vi "post.vi"(8 "error in (no error)":errorcluster, 10 "build_spec":T1, 11 "lv-build-default in":refnum<class "lv-builder.lvclass">) -> (0 "error out":errorcluster, 3 "lv-build-default out":refnum<class "lv-builder.lvclass">)   [LabVIEW 2015, in "lv-builder.lvlib" / "lv-builder.lvclass"]
uses:
  lv-builder.lvclass
  lv-build/public/_controls/build_specification.ctl
  lv-build/public/_controls/build_type.ctl
  public/_controls/configuration.ctl
  private/_controls/post_action_lvlib.ctl
  private/_controls/post_action_zip.ctl
  private/_controls/post_action_application.ctl
  private/_controls/post_action_installer.ctl
  lv-builder.lvlib
  lv-build/lv-build.lvlib
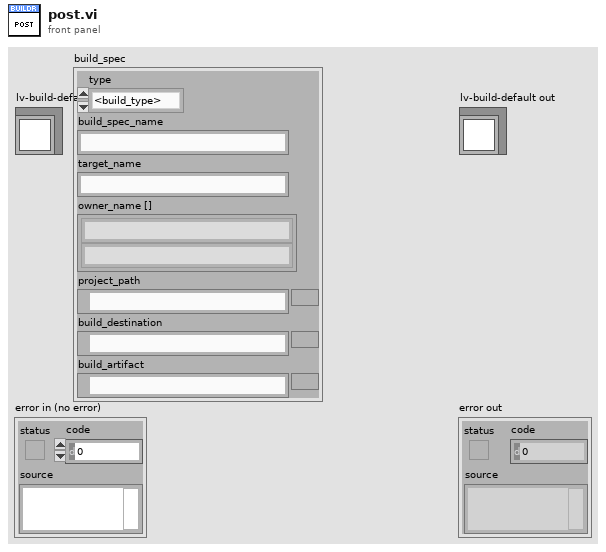
[diagram p1: front panel]
types:
  T1 = typedef "lv-build.lvlib/build_specification.ctl" = cluster{"type":T2, "build_spec_name":string, "target_name":string, "owner_name []":string[], "project_path":path, "build_destination":path, "build_artifact":path}
  T2 = typedef "lv-build.lvlib/build_type.ctl" = enum16{"<build_type>", "application_pc", "application_rt", "installer", "llb", "lvlibp", "zip", "fpga", "<null>"}
  T3 = typedef "lv-builder.lvlib/configuration.ctl" = cluster{"lvlibp_directory":string, "zip_directory":string, "lvlib_directory":string, "update_version_vi":string, "installer_post_file":string, "lvlib_post_action":u16, "installer_post_action":u16, "application_post_action":u16, "zip_post_action":u16}
  T4 = typedef "lv-builder.lvlib/post_action_lvlib.ctl" = enum16{"<lvlib_post_action>", "nothing", "move", "install", "<null>"}
  T5 = typedef "lv-builder.lvlib/post_action_zip.ctl" = enum16{"<zip_post_action>", "nothing", "move", "extract", "<null>"}
  T6 = typedef "lv-builder.lvlib/post_action_application.ctl" = enum16{"<application_post_action>", "nothing", "zip_application", "<null>"}
  T7 = typedef "lv-builder.lvlib/post_action_installer.ctl" = enum16{"<installer_post_action>", "nothing", "create_installer", "zip_installer", "create_installer_file", "<null>"}
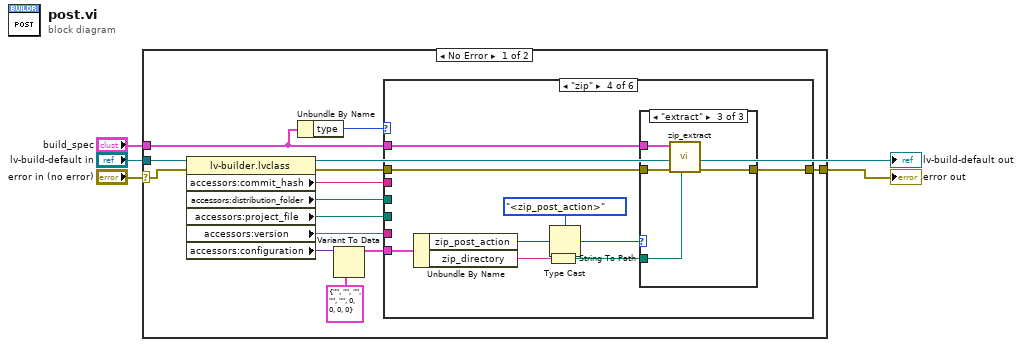
[diagram p0: block diagram]
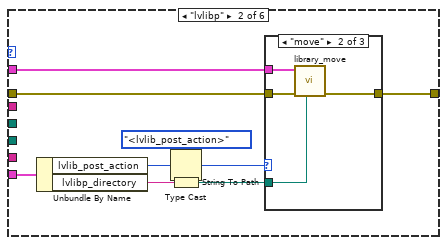
[diagram p3: hidden frame]
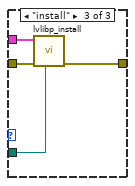
[diagram p5: hidden frame]
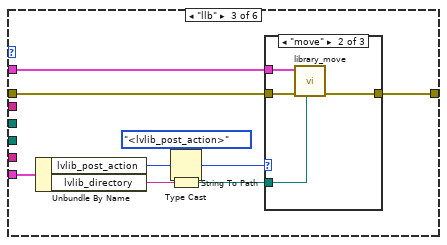
[diagram p6: hidden frame]
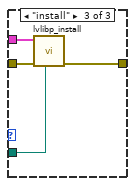
[diagram p8: hidden frame]
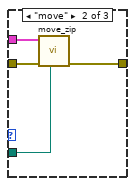
[diagram p10: hidden frame]
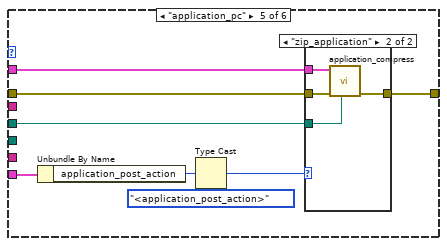
[diagram p11: hidden frame]
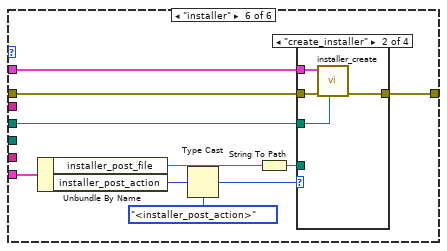
[diagram p13: hidden frame]
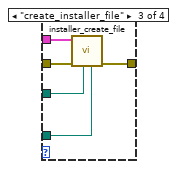
[diagram p15: hidden frame]
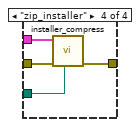
[diagram p16: hidden frame]
diagram:
  n1 = case shown="No Error" "error in (no error)" {
    selector: "error in (no error)" -> [w14 w110]
    tunnel: [w17 w110] -> w4
    tunnel: "build_spec" -> [w16 _]
    tunnel: "lv-build-default in" -> [w13 _]
    frame No Error {
      n2 = property class="lv-builder.lvclass"(reference=w13, error in=w14) -> (error out=w12:errorcluster, "accessors:commit_hash"=w11:string, "accessors:distribution_folder"=w10:path, "accessors:project_file"=w7:path, "accessors:version"=w9:string, "accessors:configuration"=w8:variant)  [unwired: 1 out]
      n3 = Unbundle By Name(w16) -> ("type"=w15:T2)
      n4 = Variant To Data(type=T3 {"lvlibp_directory"="", "zip_directory"="", "lvlib_directory"="", "update_version_vi"="", "installer_post_file"="", "lvlib_post_action"=0, "installer_post_action"=0, "application_post_action"=0, "zip_post_action"=0} ("configuration"), Variant=w8) -> (data=w5:T3)  [unwired: 1 in, 1 out]
      n5 = case shown="\"zip\"" w15 {
        tunnel: [w18 w27 w45 w63 w80 w95] -> w17
        tunnel: w16 -> [_ w26 w44 w62 w79 w94]
        tunnel: w12 -> [w18 w25 w43 w61 w78 w93]
        tunnel: w11 -> [_ _ _ _ _ _]
        tunnel: w10 -> [_ _ _ _ w73 w86]
        tunnel: w9 -> [_ _ _ _ _ _]
        tunnel: w5 -> [_ w21 w39 w57 w74 w91]
        tunnel: w7 -> [_ _ _ _ _ _]
        frame Default {
        }
        frame "lvlibp" {
          n6 = Unbundle By Name(w21) -> ("lvlib_post_action"=w23:u16, "lvlibp_directory"=w20:string)
          n7 = Type Cast(type=post_action_lvlib."<lvlib_post_action>" ("lvlib_post_action"), x=w23) -> (*(type *) &x=w22:T4)
          n8 = String To Path(string=w20) -> (path=w19:path)
          n9 = case shown="\"move\"" w22 {
            tunnel: [w28 w30 w34] -> w27
            tunnel: w26 -> [_ w31 w36]
            tunnel: w25 -> [w28 w32 w35]
            tunnel: w19 -> [_ w29 w33]
            frame Default {
            }
            frame "move" {
              n10 = call "library_move.vi"("lvlib_move_directory"=w29, "error in (no error)"=w32, "build_specifications"=w31) -> ("error out"=w30:errorcluster)  [unwired: 8 in]
            }
            frame "install" {
              n11 = call "lvlibp_install.vi"("lvlib_move_directory"=w33, "error in (no error)"=w35, "build_specifications"=w36) -> ("error out"=w34:errorcluster)  [unwired: 8 in]
            }
          }
        }
        frame "llb" {
          n12 = Unbundle By Name(w39) -> ("lvlib_post_action"=w41:u16, "lvlib_directory"=w38:string)
          n13 = Type Cast(type=post_action_lvlib."<lvlib_post_action>" ("lvlib_post_action"), x=w41) -> (*(type *) &x=w40:T4)
          n14 = String To Path(string=w38) -> (path=w37:path)
          n15 = case shown="\"move\"" w40 {
            tunnel: [w46 w48 w52] -> w45
            tunnel: w44 -> [_ w49 w54]
            tunnel: w43 -> [w46 w50 w53]
            tunnel: w37 -> [_ w47 w51]
            frame Default {
            }
            frame "move" {
              n16 = call "library_move.vi"("lvlib_move_directory"=w47, "error in (no error)"=w50, "build_specifications"=w49) -> ("error out"=w48:errorcluster)  [unwired: 8 in]
            }
            frame "install" {
              n17 = call "lvlibp_install.vi"("lvlib_move_directory"=w51, "error in (no error)"=w53, "build_specifications"=w54) -> ("error out"=w52:errorcluster)  [unwired: 8 in]
            }
          }
        }
        frame "zip" {
          n18 = Unbundle By Name(w57) -> ("zip_post_action"=w60:u16, "zip_directory"=w56:string)
          n19 = String To Path(string=w56) -> (path=w55:path)
          n20 = Type Cast(type=post_action_zip."<zip_post_action>" ("zip_post_action"), x=w60) -> (*(type *) &x=w59:T5)
          n21 = case shown="\"extract\"" w59 {
            tunnel: [w64 w66 w70] -> w63
            tunnel: w62 -> [_ w67 w71]
            tunnel: w61 -> [w64 w68 w72]
            tunnel: w55 -> [_ w65 w69]
            frame Default {
            }
            frame "move" {
              n22 = call "move_zip.vi"("zip_move_directory"=w65, "error in (no error)"=w68, "build_specifications"=w67) -> ("error out"=w66:errorcluster)  [unwired: 8 in]
            }
            frame "extract" {
              n23 = call "zip_extract.vi"("zip_extract_directory"=w69, "error in (no error)"=w72, "build_specifications"=w71) -> ("error out"=w70:errorcluster)  [unwired: 8 in]
            }
          }
        }
        frame "application_pc" {
          n24 = Unbundle By Name(w74) -> ("application_post_action"=w76:u16)
          n25 = Type Cast(type=post_action_application."<application_post_action>" ("application_post_action"), x=w76) -> (*(type *) &x=w75:T6)
          n26 = case shown="\"zip_application\"" w75 {
            tunnel: [w81 w83] -> w80
            tunnel: w79 -> [_ w85]
            tunnel: w78 -> [w81 w84]
            tunnel: w73 -> [_ w82]
            frame "nothing", Default {
            }
            frame "zip_application" {
              n27 = call "application_compress.vi"("distribution_folder"=w82, "error in (no error)"=w84, "build_specifications"=w85) -> ("error out"=w83:errorcluster)  [unwired: 8 in]
            }
          }
        }
        frame "installer" {
          n28 = Unbundle By Name(w91) -> ("installer_post_file"=w87:string, "installer_post_action"=w88:u16)
          n29 = Type Cast(type=post_action_installer."<installer_post_action>" ("installer_post_action"), x=w88) -> (*(type *) &x=w89:T7)
          n30 = String To Path(string=w87) -> (path=w92:path)
          n31 = case shown="\"create_installer\"" w89 {
            tunnel: [w96 w98 w103 w107] -> w95
            tunnel: w94 -> [_ w99 w104 w109]
            tunnel: w93 -> [w96 w100 w105 w108]
            tunnel: w92 -> [_ _ w101 _]
            tunnel: w86 -> [_ w97 w102 w106]
            frame "nothing", Default {
            }
            frame "create_installer" {
              n32 = call "installer_create.vi"("distribution_folder"=w97, "error in (no error)"=w100, "build_specifications"=w99) -> ("error out"=w98:errorcluster)  [unwired: 8 in]
            }
            frame "create_installer_file" {
              n33 = call "installer_create_file.vi"("special_file"=w101, "distribution_folder"=w102, "error in (no error)"=w105, "build_specifications"=w104) -> ("error out"=w103:errorcluster)  [unwired: 7 in]
            }
            frame "zip_installer" {
              n34 = call "installer_compress.vi"("distribution_folder"=w106, "error in (no error)"=w108, "build_specifications"=w109) -> ("error out"=w107:errorcluster)  [unwired: 8 in]
            }
          }
        }
      }
    }
    frame Error {
    }
  }
  "error out" <- w4
  "lv-build-default out" <- "lv-build-default in"
